vi "Xml_Load_Spectrum.vi"(7 "Version String":string, 8 "error in (no error)":errorcluster, 10 "XML Path":path=path "D:/TEST.xml", 11 "Refnum Clust":refnum<vi>) -> (0 "error out":errorcluster)   [LabVIEW 2020]
uses:
  controls/SPECTRUM.ctl
panel:
  in  "SPECTRUM":T1={"Day Path"=path "D:/PIRENEA/DATA/2016/data_2016_01_01", "Spectrum Name"="2016_01_01_000.A00", "Accumulated"=FALSE, "Stored in Database"=FALSE, "From a Set of"=1, "Quality Flag"="Optimal"}
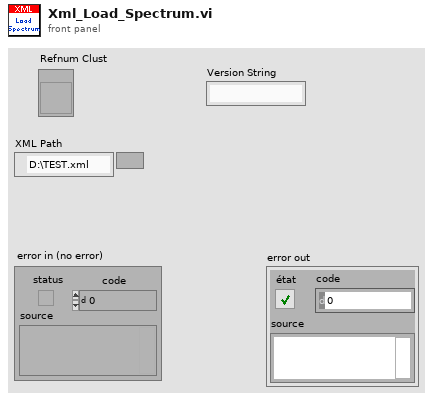
[diagram p1: front panel]
types:
  T1 = typedef "SPECTRUM.ctl" = cluster{"Day Path":path, "Spectrum Name":string, "Accumulated":bool, "Stored in Database":bool, "From a Set of":i16, "Quality Flag":string}
  T2 = cluster{"Path of the Day":path, "Spectrum Name":string, "Accumulated":bool, "Stored in Database":bool, "Record Number":i16, "Quality Flag":string}
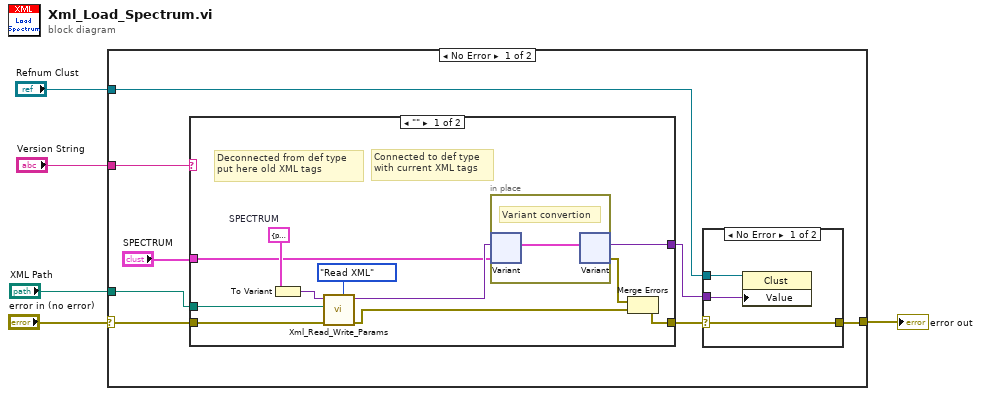
[diagram p0: block diagram]
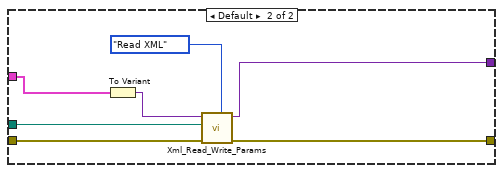
[diagram p2: hidden frame]
diagram:
  n1 = case shown="No Error" "error in (no error)" {
    selector: "error in (no error)" -> [w12 w37]
    tunnel: [w7 w37] -> w4
    tunnel: "XML Path" -> [w11 _]
    tunnel: "Version String" -> [w13 _]
    tunnel: "Refnum Clust" -> [w8 _]
    frame No Error {
      n2 = case shown="\"\"" w13 {
        tunnel: w12 -> [w22 w30]
        tunnel: [w15 w27] -> w10
        tunnel: [w18 w28] -> w9
        tunnel: w11 -> [w21 w29]
        tunnel: "SPECTRUM" -> [w14 w26]
        frame "" {
          w19 = T2 {"Path of the Day"=path "D:/PIRENEA/DATA/2016/data_2016_01_01", "Spectrum Name"="", "Accumulated"=FALSE, "Stored in Database"=FALSE, "Record Number"=0, "Quality Flag"="Optimal"}  # SPECTRUM
          # "Connected to def type\nwith current XML tags"
          # "Deconnected from def type\nput here old XML tags"
          n3 = To Variant(anything=w19) -> (Variant=w23:variant)
          n4 = call "Xml_Read_Write_Params.vi"("Variant"=w23, "XML Path"=w21, "error in (no error)"=w22, "Command"=enum16{"Read XML", "Set", "Get", "Write XML"}."Read XML") -> ("Variant Output"=w20:variant, "error out"=w16:errorcluster)  [unwired: 3 in, 1 out]
          n5 = in-place "Structure Élément en place" {
            # "Variant convertion"
            n6 = in-place-variant #1(w20, w14) -> (w25:T1)  [unwired: 1 out]
            n7 = in-place-variant #1(w25) -> (w18:variant, w17:errorcluster)
          }
          n8 = Merge Errors(w17, w16) -> (w15:errorcluster)
        }
        frame Default {
          n9 = To Variant(anything=w26) -> (Variant=w31:variant)
          n10 = call "Xml_Read_Write_Params.vi"("Variant"=w31, "XML Path"=w29, "error in (no error)"=w30, "Command"=enum16{"Read XML", "Set", "Get", "Write XML"}."Read XML") -> ("Variant Output"=w28:variant, "error out"=w27:errorcluster)  [unwired: 3 in, 1 out]
        }
      }
      n11 = case shown="No Error" w10 {
        selector: w10 -> [w33 w36]
        tunnel: w9 -> [w35 _]
        tunnel: w8 -> [w34 _]
        tunnel: [w33 w36] -> w7
        frame No Error {
          n12 = property class="Clust"(reference=w34, "Value"=w35) -> ()  [unwired: 1 in, 2 out]
        }
        frame Error {
        }
      }
    }
    frame Error {
    }
  }
  "error out" <- w4
